vi "Set Car Position Changed Event.vi"(7 "Name":string, 10 "Format":string, 11 "Station":string) -> (3 "Car Position Changed out":refnum<class "Car Position Changed.lvclass">)   [LabVIEW 2016, in "CLD Exam - Car Wash.lvlib" / "Car Position Changed.lvclass"]
uses:
  Car Position Changed.lvclass
  D:/Repos/Stream/software/Mediator/Classes/Message Interface/Message Interface.lvclass
  Car Position Changed.lvclass/Car Position Changed.ctl
  Mediator/Classes/Message Interface/Message Interface.lvclass
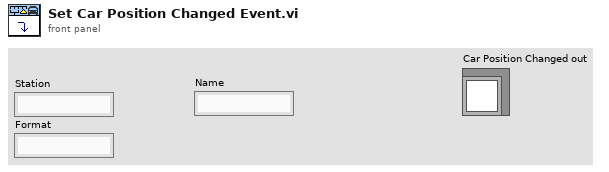
[diagram p1: front panel]
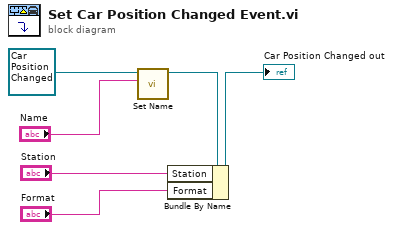
[diagram p0: block diagram]
diagram:
  n1 = call "Set Name.vi"("Name"="Name", "Message Interface in"=refnum<class "Car Position Changed.lvclass"> refnum ("Car Position Changed in")) -> ("Message Interface out"=w6:refnum<class "Car Position Changed.lvclass">)  [unwired: 8 in, 1 out]
  n2 = Bundle By Name(cluster=w6, "Station"="Station", "Format"="Format") -> (→"Car Position Changed out":refnum<class "Car Position Changed.lvclass">)
